vi "PFI-28000-Utils_Query.vi"(0 "VISA resource name":refnum<visa-resource-name>, 5 "Command":string, 11 "error in (no error)":errorcluster) -> (4 "VISA resource name out":refnum<visa-resource-name>, 6 "Return":string, 15 "error out":errorcluster)   [LabVIEW 2017, in "PFI-28000-Utils.lvlib"]
uses:
  PFI-28000-Utils.lvlib
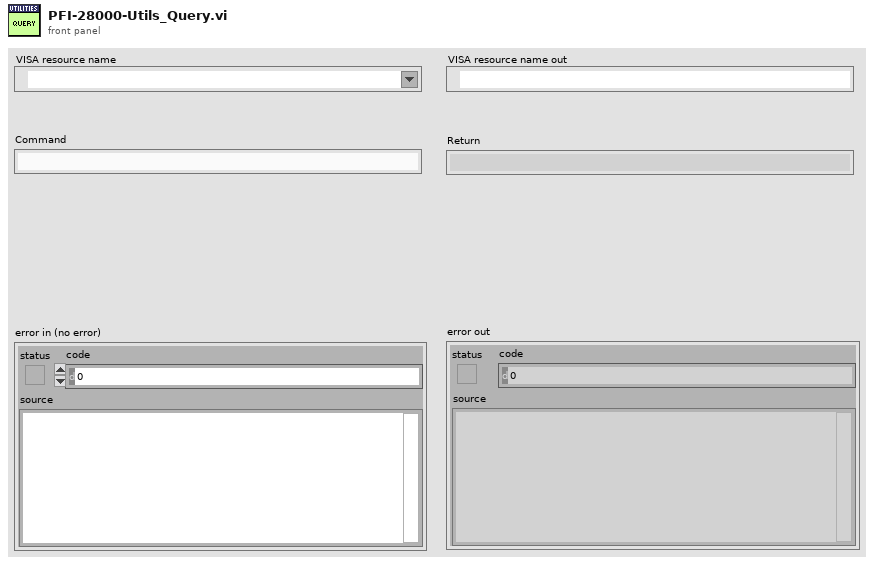
[diagram p1: front panel]
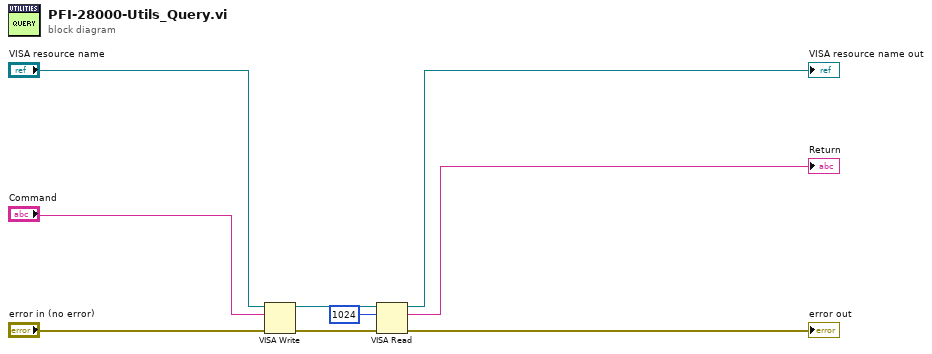
[diagram p0: block diagram]
diagram:
  n1 = VISA Write(VISA resource name="VISA resource name", write buffer="Command", error in (no error)="error in (no error)") -> (VISA resource name out=w5:refnum<visa-resource-name>, error out=w7:errorcluster)  [unwired: 1 out]
  n2 = VISA Read(VISA resource name=w5, byte count=u32 1024, error in (no error)=w7) -> (VISA resource name out=→"VISA resource name out":refnum<visa-resource-name>, read buffer=→"Return":string, error out=→"error out":errorcluster)  [unwired: 1 out]
